vi "_Destroy.vi"(8 "error in (no error)":errorcluster, 11 "Reader in":refnum<class "Reader.lvclass">) -> (0 "error out":errorcluster, 2 "Finalized Readable":refnum<class "Readable.lvclass">)   [LabVIEW 2009, in "Reader.lvclass"]
uses:
  Reader.lvclass
  Instruments/Utility Classes/Readable/Readable.lvclass
  Reader.lvclass/Reader.ctl
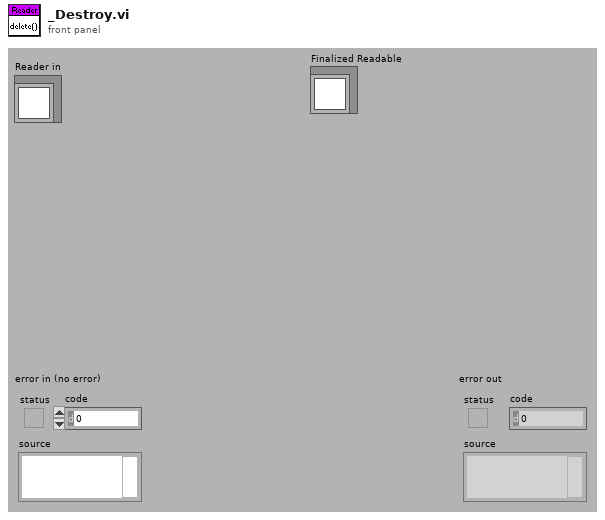
[diagram p1: front panel]
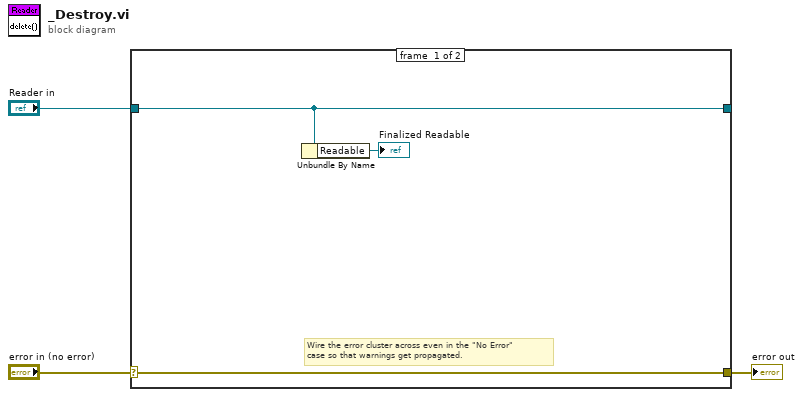
[diagram p0: block diagram]
diagram:
  n1 = case shown="No Error" "error in (no error)" {
    selector: "error in (no error)" -> [w6 w8]
    tunnel: [w6 w8] -> w2
    tunnel: [w5 w7] -> _
    tunnel: "Reader in" -> [w5 w7]
    frame #0 {
      # "Wire the error cluster across even in the \"No Error\"\ncase so that warnings get propagated."
      n2 = Unbundle By Name(w5) -> ("Readable"=→"Finalized Readable":refnum<class "Readable.lvclass">)
    }
    frame #1 {
    }
  }
  "error out" <- w2
